vi "DataloggingTEST.vi"() -> ()   [LabVIEW 2017]
uses:
  <vilib>/Platform/TimedLoop/XDataNode/timing_clust.ctl
  <vilib>/Platform/TimedLoop/XDataNode/nitl_modes.ctl
  <vilib>/Platform/TimedLoop/XDataNode/wakeup.ctl
  <vilib>/platform/TimedLoop/XDataNode/XDataNode.xnode
  <vilib>/Platform/TimedLoop/XDataNode/XDNodeRunTimeDep.lvlib
panel:
  in  "Frequency (Hz)":dbl=100.0
  in  "Stop":bool
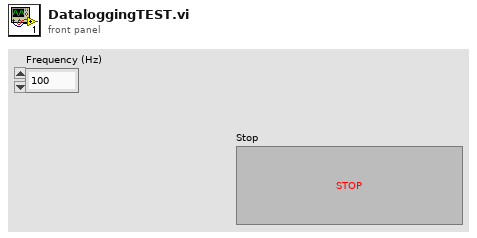
[diagram p1: front panel]
types:
  T1 = enum16{"open", "open or create", "create or replace", "create", "open (read-only)"}
  T2 = typedef "XDNodeRunTimeDep.lvlib/timing_clust.ctl" = cluster{"Expected End [f-1]":u64, "Actual End [f-1]":u64, "Finished Late? [f-1]":bool, "Expected End [i-1]":u64, "Actual End [i-1]":u64, "Finished Late? [i-1]":bool, "Expected Start [i]":u64, "Actual Start [i]":u64, "Expected Start [f]":u64, "Actual Start [f]":u64, "Source Name":string, "Structure Name":string, "Period":i64, "Deadline":i64, "Offset":i64, "Start":i64, "Priority":i32, "Timeout":i32, "Mode":T3, "Wakeup Reason":T4, "Error":errorcluster, "Source Type":string, "Secondary Source Type":string, "Global End Time":u64, "Global Start Time":u64, "Frame Duration":u64, "Iteration Duration":u64, "Assigned CPU":i32, "I/O Scan Engine Mode":u32}
  T3 = typedef "XDNodeRunTimeDep.lvlib/nitl_modes.ctl" = enum32{"No Change", "Process missed periods, maintain original phase", "Discard missed periods, maintain original phase", "Process missed periods, ignore original phase", "Discard missed periods, ignore original phase"}
  T4 = typedef "XDNodeRunTimeDep.lvlib/wakeup.ctl" = enum32{"Normal", "Aborted", "Asynchronous wakeup", "Timing source error", "Timed loop error", "Timeout"}
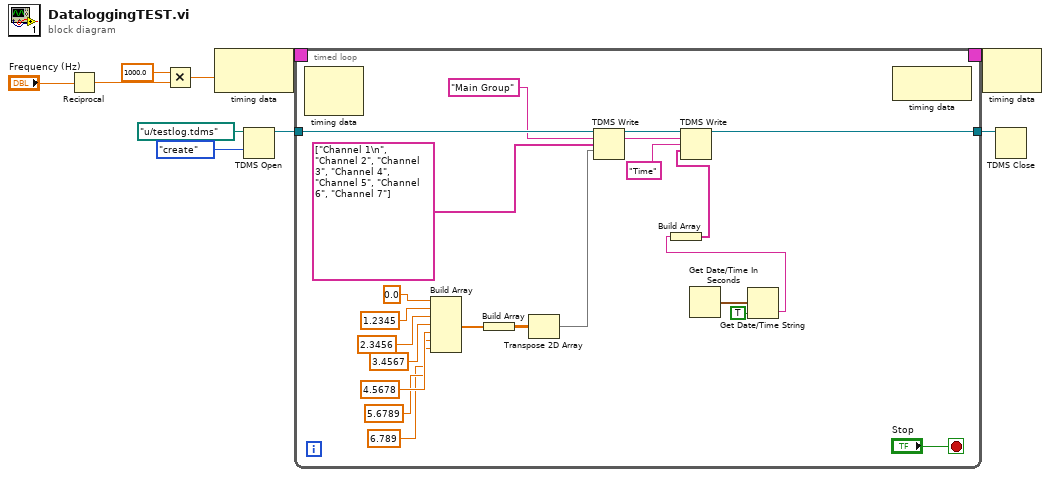
[diagram p0: block diagram]
diagram:
  n1 = Reciprocal(x="Frequency (Hz)") -> (1/x=w2:dbl)
  n2 = Multiply(x=1000.0, y=w2) -> (x*y=w4:dbl)
  n3 = node-c288(w4) -> (w10:T2)
  n4 = TDMS Open(10:T1."create" ("operation (0:open)"), 11:path "u:/testlog.tdms" ("file path")) -> (3:w6:refnum<k34>)  [unwired: 5 in, 1 out]
  n5 = timed-loop {
    timing: w10 -> [_]
    timing-out: [_] -> w9
    tunnel: [w29] -> w8
    tunnel: w6 -> [w32]
    stop <- "Stop" stop-if-true
    n6 = node-c288() -> ()  [unwired: 1 in, 2 out]
    n7 = Build Array(0.0, 1.2345, 2.3456, 3.4567, 4.5678, 5.6789, 6.789) -> (w13:dbl[])
    n8 = Build Array(w13) -> (w12:dbl[][])
    n9 = Transpose 2D Array(2D array=w12) -> (transposed array=w11:dbl[][])
    n10 = TDMS Write(0:w32, 5:"Main Group" ("group name in (Untitled)"), 7:string[] ["Channel 1\n", "Channel 2", "Channel 3", "Channel 4", "Channel 5", "Channel 6", "Channel 7"] ("channel name(s) in (Untitled)"), 9:w11) -> (4:w30:refnum<k34>, 6:w22:string)  [unwired: 2 in, 2 out]
    n11 = Get Date/Time In Seconds() -> (seconds since 1Jan1904=w26:timestamp)
    n12 = Get Date/Time String(seconds (now)=w26, want seconds? (F)=TRUE) -> (time string=w24:string)  [unwired: 1 in, 1 out]
    n13 = Build Array(w24) -> (w27:string[])
    n14 = TDMS Write(0:w30, 5:w22, 7:"Time", 9:w27) -> (4:w29:refnum<k34>)  [unwired: 2 in, 3 out]
    n15 = node-c288() -> ()  [unwired: 1 in, 1 out]
  }
  n16 = node-c288(w9) -> ()  [unwired: 1 out]
  n17 = TDMS Close(11:w8) -> ()  [unwired: 1 in, 2 out]
